vi "Write_to_file_example.vi"() -> ()   [LabVIEW 2022 SP3]
panel:
  out "EOF?":bool
  in  "Start to read":bool
  in  "Start to write":bool
  out "Waveform \"Read\"":dynamicdata(graph)
  in  "Frequency":dbl=1.0
  out "Waveform \"Write\"":dynamicdata(graph)
  in  "file path":path
  in  "stop":bool
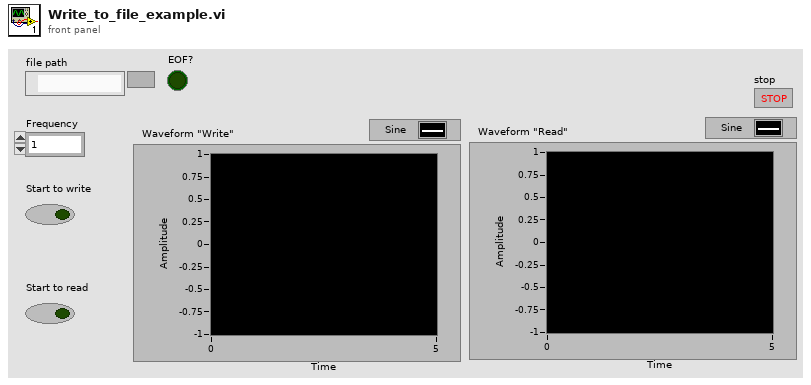
[diagram p1: front panel]
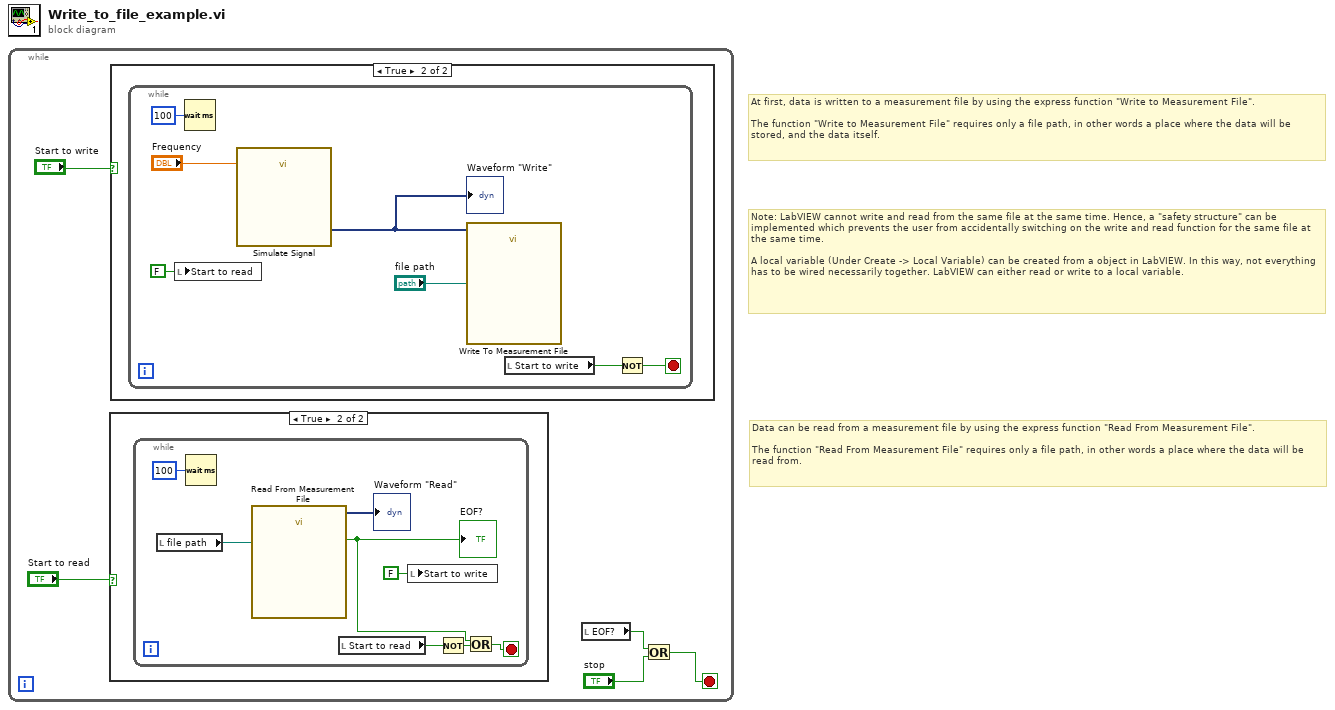
[diagram p0: block diagram]
diagram:
  # "Note: LabVIEW cannot write and read from the same file at the same time. Hence, a \"safety structure\" can be implemented which prevents the user from accidentally switching on the write and read function for the same file at the same time.\n\nA local variable (Under Create -> Local Variable) can be created from a object in LabVIEW. In this way, not everything has to be wired necessarily together. LabVIEW can either read or write to a local variable."
  # "Data can be read from a measurement file by using the express function \"Read From Measurement File\".\n\nThe function \"Read From Measurement File\" requires only a file path, in other words a place where the data will be read from."
  # "At first, data is written to a measurement file by using the express function \"Write to Measurement File\".\n\nThe function \"Write to Measurement File\" requires only a file path, in other words a place where the data will be stored, and the data itself."
  n1 = while {
    stop <- w1 stop-if-true
    n2 = case shown="True" "Start to read" {
      frame False {
      }
      frame True {
        n3 = while {
          stop <- w15 stop-if-true
          n4 = local read "file path"() -> (w19:path)
          n5 = Wait (ms)(milliseconds to wait=u32 100) -> ()  [unwired: 1 out]
          n6 = call "Read From Measurement File"("Filename"=w19) -> ("Signals"=→"Waveform \"Read\"":dynamicdata, "EOF?"=w13:bool)  [unwired: 5 in, 4 out]
          "EOF?" <- w13
          n7 = local read "Start to read"() -> (w18:bool)
          n8 = local write "Start to write"(FALSE ("Start to write")) -> ()
          n9 = Not(x=w18) -> (.not. x?=w14:bool)
          n10 = Or(x=w13, y=w14) -> (x .or. y?=w15:bool)
        }
      }
    }
    n11 = case shown="True" "Start to write" {
      frame False {
      }
      frame True {
        n12 = while {
          stop <- w8 stop-if-true
          n13 = local write "Start to read"(FALSE ("Start to read")) -> ()
          n14 = Wait (ms)(milliseconds to wait=u32 100) -> ()  [unwired: 1 out]
          n15 = call "Simulate Signal"("Frequency"="Frequency") -> ("Sine"=w10:dynamicdata)  [unwired: 13 in, 1 out]
          "Waveform \"Write\"" <- w10
          n16 = call "Write To Measurement File"("Signals"=w10, "Filename"="file path") -> ()  [unwired: 15 in, 3 out]
          n17 = local read "Start to write"() -> (w7:bool)
          n18 = Not(x=w7) -> (.not. x?=w8:bool)
        }
      }
    }
    n19 = local read "EOF?"() -> (w3:bool)
    n20 = Or(x=w3, y="stop") -> (x .or. y?=w1:bool)
  }
